vi "AdaptToInputs.vi"(3 "Term Types":T1[](array[typedef]), 4 "XRef":refnum<vi>, 5 "State In":T4={"Input Type"=variant(dbl 0.0), "Error"={"status"=FALSE, "code"=0, "source"=""}}) -> (0 "Reply":string[](array[string]), 2 "State Out":T4={"Input Type"=variant(dbl 0.0), "Error"={"status"=FALSE, "code"=0, "source"=""}})   [LabVIEW 2015, in "Destroy-Signals.xnode"]
doc: "This ability VI is called by LabVIEW during type propagation so that your XNode may adapt itself to new input types. Term Types is an array of pairs of current Term IDs and the type descriptors corresponding to them. The type descriptors are taken from the signal connected to the terminal. Unwired terminals are not included in the array. Use Reply to inform LabVIEW of any actions it needs to take.\n\nDefault behavior: None.\n\nThis ability does not provide UI and OS messages are not handled."
uses:
  Destroy-Signals.xnode
  State.ctl
  <vilib>/XNodeSupport/XNodeTermTypeIDPair.ctl
  <vilib>/XNodeSupport/XNodeType.ctl
  <vilib>/XNodeSupport/XNodeString.ctl
  <vilib>/Erdos Miller/LV-Scripting/LV-Scripting.lvlib
  <vilib>/XNodeSupport/NI_XNodeSupport.lvlib
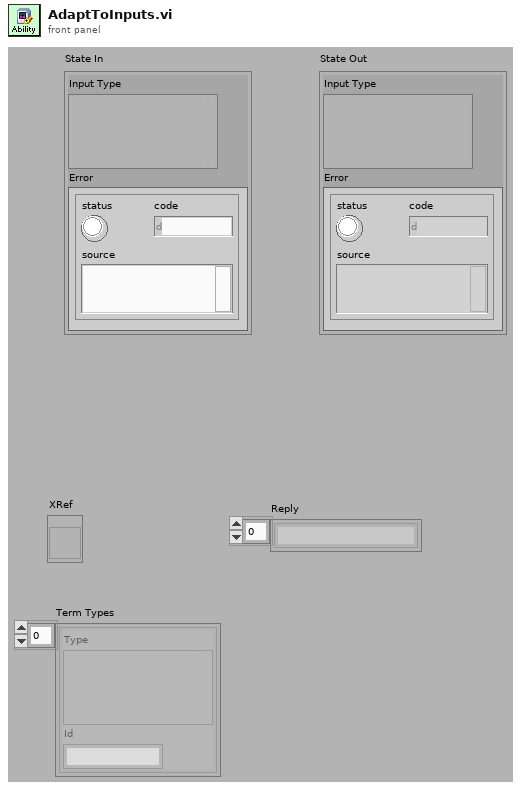
[diagram p1: front panel]
types:
  T1 = typedef "NI_XNodeSupport.lvlib/XNodeTermTypeIDPair.ctl" = cluster{"Type":T2, "Id":T3}
  T2 = typedef "NI_XNodeSupport.lvlib/XNodeType.ctl" = variant
  T3 = typedef "NI_XNodeSupport.lvlib/XNodeString.ctl" = string
  T4 = typedef "Destroy-Signals.xnode/State.ctl" = cluster{"Input Type":variant, "Error":errorcluster}
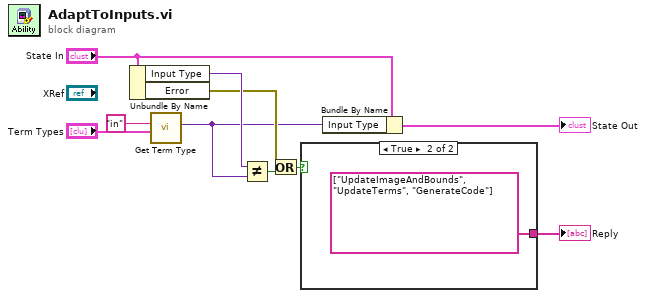
[diagram p0: block diagram]
diagram:
  n1 = Unbundle By Name("State In") -> ("Input Type"=w10:variant, "Error"=w5:errorcluster)
  n2 = call <vilib>:"Get Term Type.vi"("Term Types"="Term Types", "ID"="in" ("Search ID")) -> ("Type"=w1:variant)  [unwired: 9 in]
  n3 = Not Equal?(x=w10, y=w1) -> (x != y?=w6:bool)
  n4 = Or(x=w5, y=w6) -> (x .or. y?=w4:bool)
  n5 = case shown="True" w4 {
    tunnel: [_ string[] ["UpdateImageAndBounds", "UpdateTerms", "GenerateCode"] ("Reply")] -> w7
    frame False {
    }
    frame True {
    }
  }
  "Reply" <- w7
  n6 = Bundle By Name(cluster="State In", "Input Type"=w1) -> (→"State Out":T4)
